vi "register.public_lua.vi"(5 "LuaVIEW reference":T1) -> (15 "error out":errorcluster)   [LabVIEW 2012]
doc: "Registers a LuaVIEW function VI with the public function registry. The functions in the public registry are set when a script is started. Thus, the function will be available to subsequently started scripts yet remain invisible to already running scripts (including the script that called this registration function). When a VI with the same name is already loaded in memory, that VI will be registered. If the path is relative, the function VI is assumed to be located relative to the resource base path. If the application is built and the function VI could not be located at the specified path, the VIs built into the application executable will be searched. The registered function remains loaded until the public registry is cleaned up.\nParameters:\nstr:path, path to the function VI.\nErrors:\nFunction name invalid.\nCould not load function VI.\nFunction VI has an invalid connector pane.\nFunction improperly documented."
uses:
  typedefs/t_LuaVIEW Reference.ctl
  subvis/private/LuaVIEW Pull (path).vi
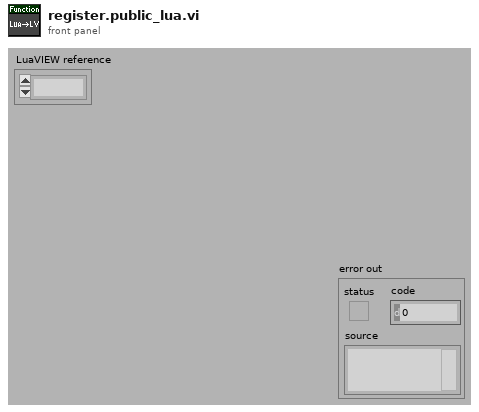
[diagram p1: front panel]
types:
  T1 = typedef "t_LuaVIEW Reference.ctl" = refnum<k1>
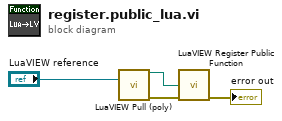
[diagram p0: block diagram]
diagram:
  n1 = call-poly "LuaVIEW Pull (poly).vi"("LuaVIEW reference in"="LuaVIEW reference") -> ("path"=w1:path, "error out"=w2:errorcluster)  [unwired: 12 in, 1 out]
  n2 = call "LuaVIEW Register Public Function.vi"("function VI path"=w1, "error in (no error)"=w2) -> ("error out"=→"error out":errorcluster)  [unwired: 13 in]
